vi "Builder.vi"(8 "error in":errorcluster, 10 "Index":i32, 11 "Builder in":refnum<class "Builder.lvclass">) -> (0 "error out":errorcluster, 2 "Generated files":path[](array[path]), 3 "Builder out":refnum<class "Builder.lvclass">)   [LabVIEW 2021, in "App-Builder Library.lvlib" / "Builder.lvclass"]
uses:
  Builder.lvclass
  Builder.lvclass/Builder.ctl
  <vilib>/AppBuilder/AB_API_Simple/Build (path).vi
  <vilib>/AppBuilder/AB_API_Simple/NI_App_Builder_API.lvlib
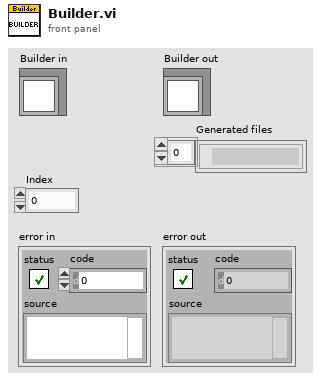
[diagram p1: front panel]
types:
  T1 = typedef "App-Builder Library.lvlib/Builder.lvclass/Build specification.ctl" = cluster{"target name":string, "Build specification":string, "Project Path":path, "Build Object type":T2}
  T2 = typedef "App-Builder Library.lvlib/Builder.lvclass/Build object type.ctl" = enum16{"EXE", "RT EXE", "Deployable Packed"}
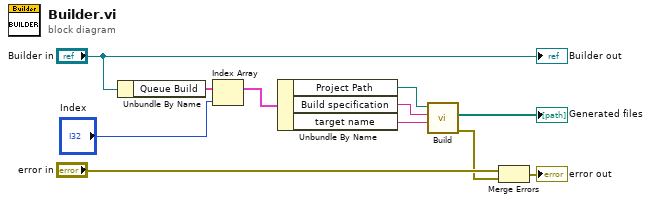
[diagram p0: block diagram]
diagram:
  n1 = Unbundle By Name("Builder in") -> ("Queue Build"=w6:T1[])
  n2 = Index Array(array=w6, index="Index") -> (element=w5:T1)
  n3 = Unbundle By Name(w5) -> ("Project Path"=w1:path, "Build specification"=w2:string, "target name"=w3:string)
  n4 = call-poly <vilib>:"Build.vi"("Name of target (My Computer)"=w3, "Name of build specification (if empty: build all)"=w2, "Path to project"=w1) -> ("error out"=w7:errorcluster, "Generated files"=→"Generated files":path[])  [unwired: 7 in]
  n5 = Merge Errors("error in", w7) -> (→"error out":errorcluster)
  "Builder out" <- "Builder in"
